vi "Adaptive Filter sim_edit_JMS.vi"() -> ()   [LabVIEW 2013]
uses:
  <vilib>/Utility/file.llb/Read From Spreadsheet File (I64).vi
panel:
  in  "Rescale":bool
  in  "Decimate":bool
  out "Gradients":dbl[][](graph)
  in  "Filter":bool
  in  "Filter Size":i32=100
  out "Weights":dbl[][](graph)
  out "Taps":dbl[][](graph)
  in  "Beta":fxp<+/-,32,-16>=1.000088900582341e-11
  out "ECG Data":dbl[][](graph)
  in  "File Path Control":path=path "C:/Users/pursley/Documents/Projects/NHLBI/Lederman/Testing/2014-03-21/FL1.txt"
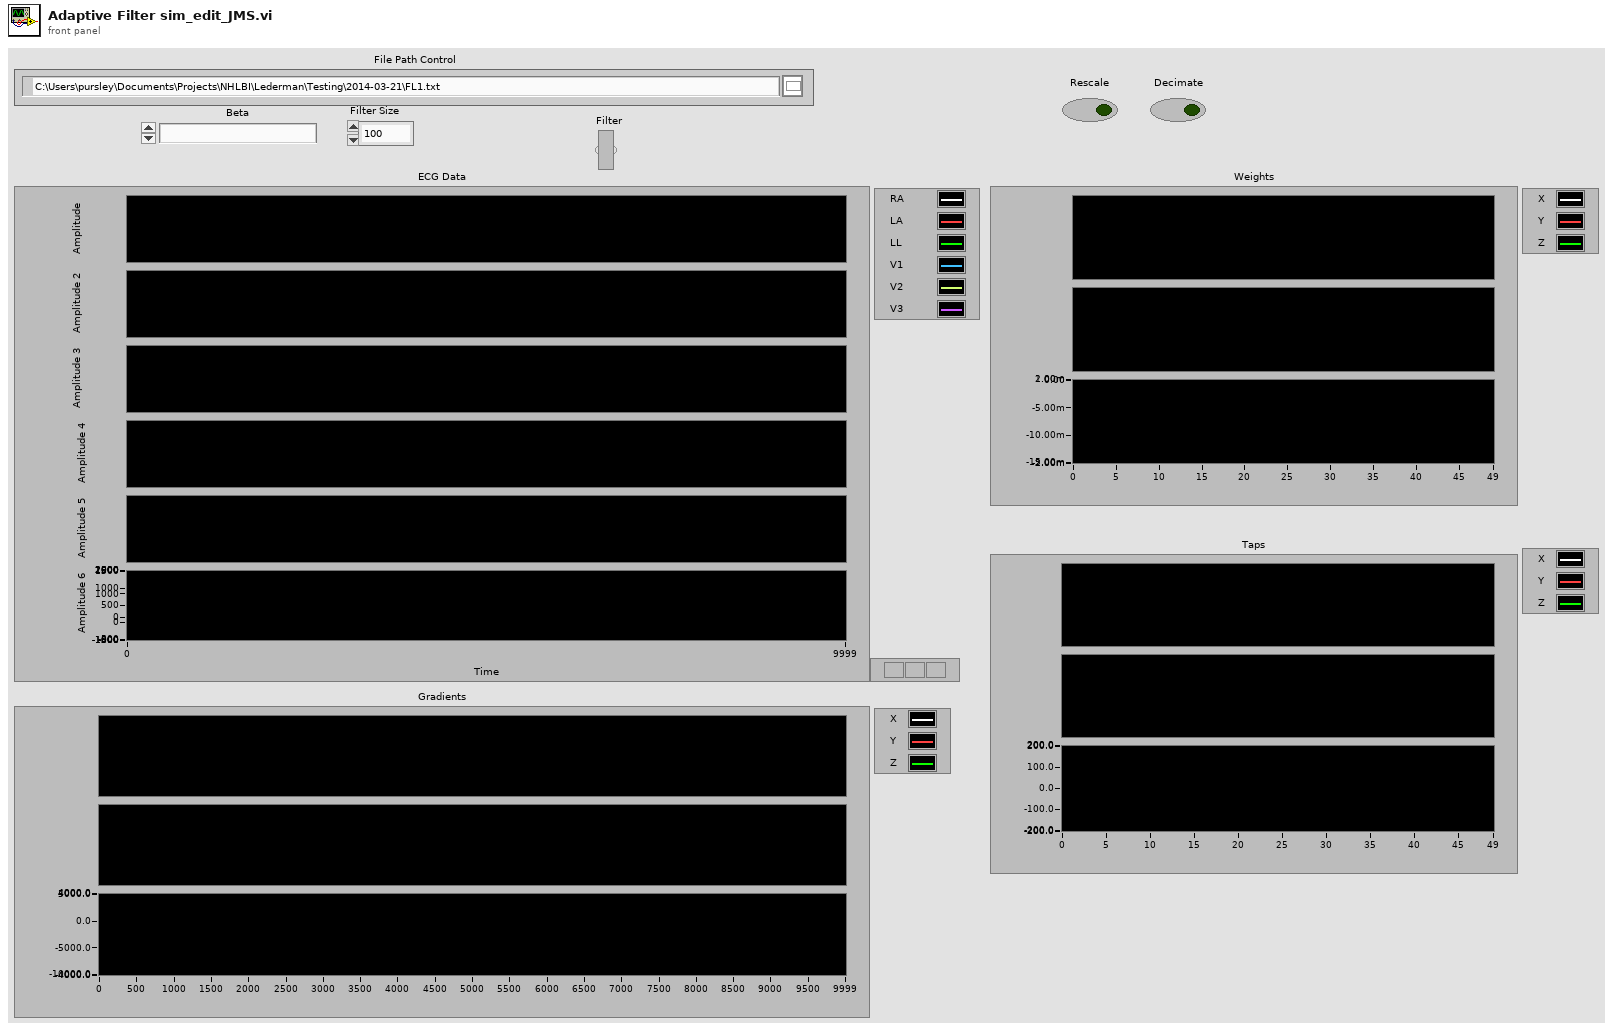
[diagram p1: front panel]
types:
  T1 = cluster{"fixed-point type":fxp<+/-,16,16>, "fixed-point type":fxp<+/-,16,16>, "fixed-point type":fxp<+/-,16,16>}
  T2 = cluster{"fixed-point type":dbl, "fixed-point type":dbl, "fixed-point type":dbl}
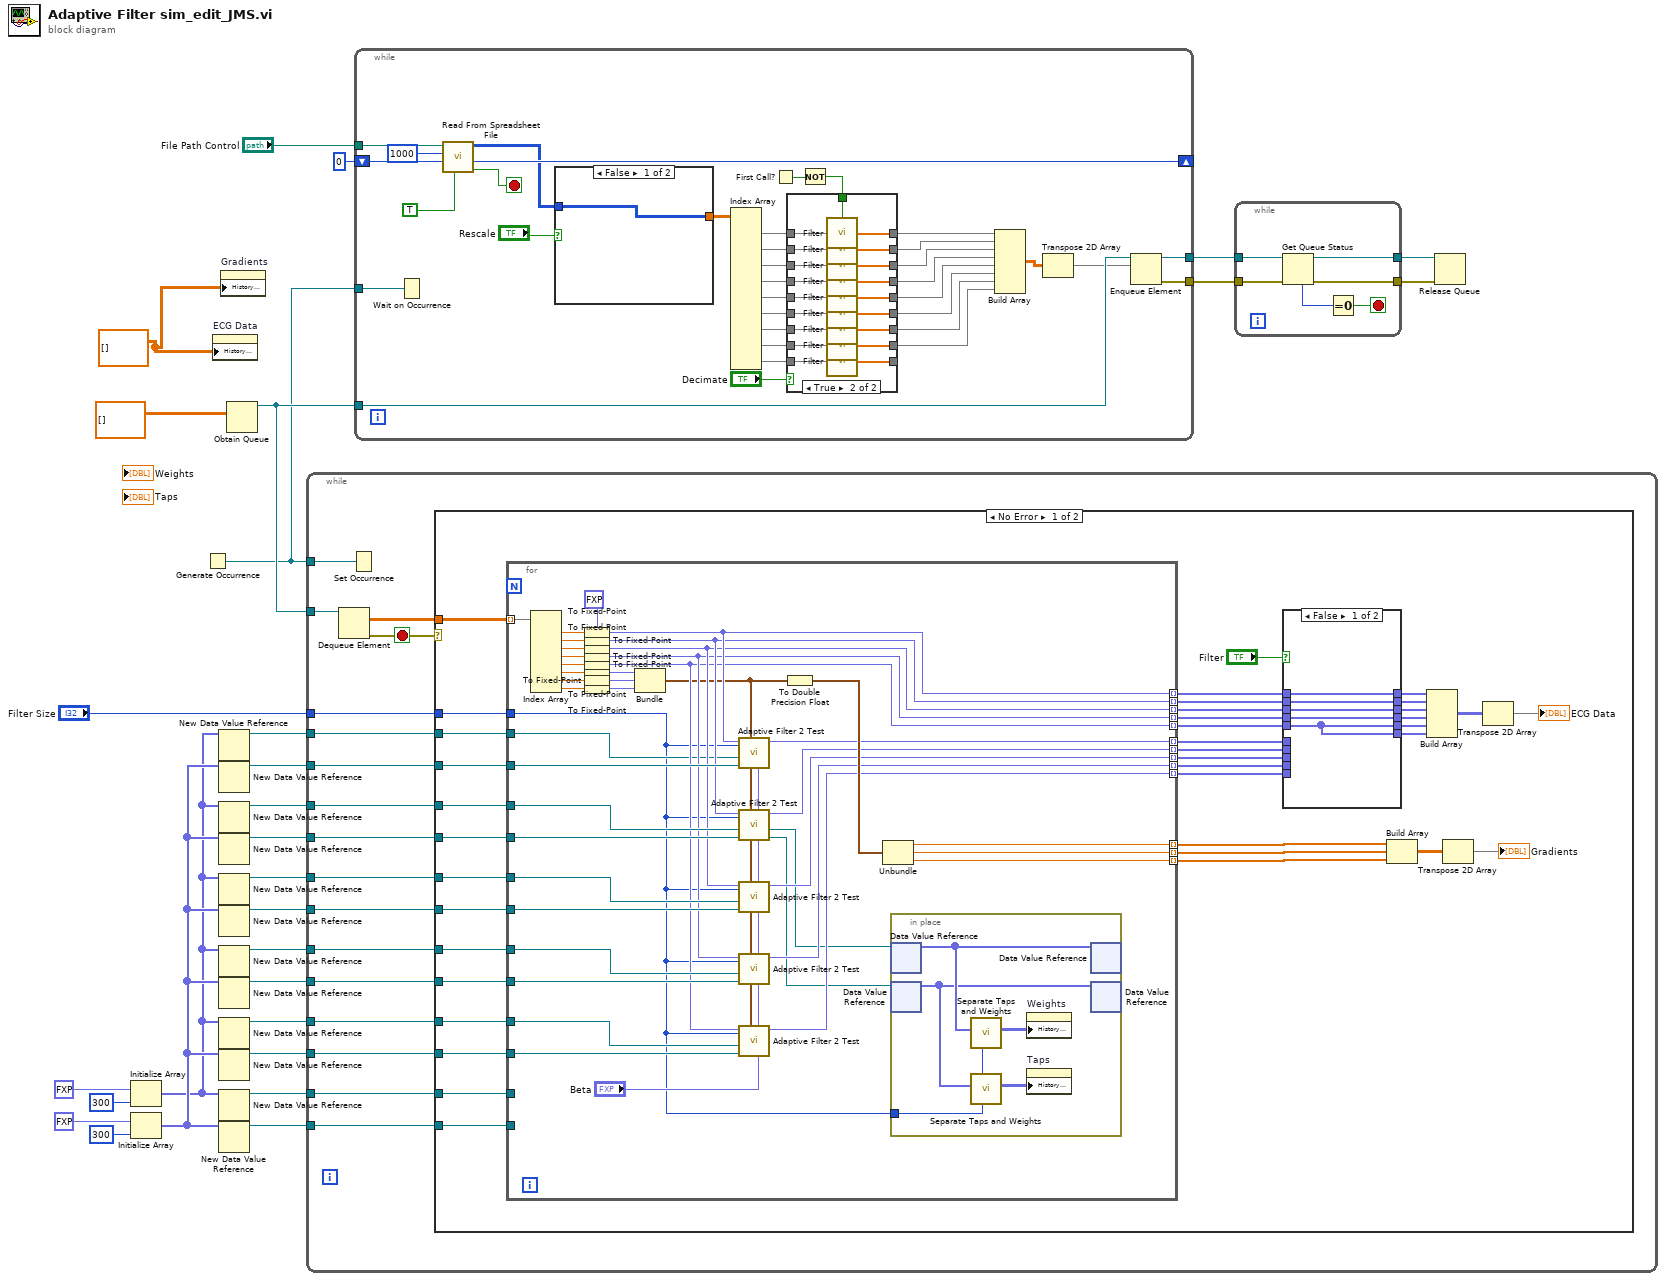
[diagram p0: block diagram]
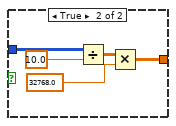
[diagram p4: hidden frame]
diagram:
  w1 = dbl[][] [] ("History Data")
  n1 = Initialize Array(fxp<+/-,24,8> 0.0 ("Z"), 300 ("dimension size")) -> (w8:fxp<+/-,24,8>[])
  n2 = Initialize Array(fxp<+/-,16,16> 0.0 ("Z"), 300 ("dimension size")) -> (w11:fxp<+/-,16,16>[])
  n3 = Generate Occurrence() -> (w2:refnum<k4>)
  n4 = property on="ECG Data" class="WFChart (strict)"("History Data"=w1) -> ()  [unwired: 2 in, 2 out]
  n5 = New Data Value Reference(data value=w8) -> (data value reference=w25:refnum<data-value>)  [unwired: 1 in, 1 out]
  n6 = New Data Value Reference(data value=w11) -> (data value reference=w24:refnum<data-value>)  [unwired: 1 in, 1 out]
  n7 = New Data Value Reference(data value=w8) -> (data value reference=w22:refnum<data-value>)  [unwired: 1 in, 1 out]
  n8 = New Data Value Reference(data value=w11) -> (data value reference=w23:refnum<data-value>)  [unwired: 1 in, 1 out]
  n9 = New Data Value Reference(data value=w8) -> (data value reference=w20:refnum<data-value>)  [unwired: 1 in, 1 out]
  n10 = New Data Value Reference(data value=w11) -> (data value reference=w21:refnum<data-value>)  [unwired: 1 in, 1 out]
  n11 = New Data Value Reference(data value=w8) -> (data value reference=w18:refnum<data-value>)  [unwired: 1 in, 1 out]
  n12 = New Data Value Reference(data value=w11) -> (data value reference=w19:refnum<data-value>)  [unwired: 1 in, 1 out]
  n13 = New Data Value Reference(data value=w8) -> (data value reference=w16:refnum<data-value>)  [unwired: 1 in, 1 out]
  n14 = New Data Value Reference(data value=w11) -> (data value reference=w17:refnum<data-value>)  [unwired: 1 in, 1 out]
  n15 = New Data Value Reference(data value=w8) -> (data value reference=w14:refnum<data-value>)  [unwired: 1 in, 1 out]
  n16 = New Data Value Reference(data value=w11) -> (data value reference=w15:refnum<data-value>)  [unwired: 1 in, 1 out]
  n17 = property on="Gradients" class="WFChart (strict)"("History Data"=w1) -> ()  [unwired: 2 in, 2 out]
  n18 = Obtain Queue(element data type=dbl[][] [] ("History Data")) -> (queue out=w26:refnum<queue>)  [unwired: 4 in, 2 out]
  n19 = while {
    tunnel: w26 -> [w30]
    tunnel: w25 -> [w44]
    tunnel: w24 -> [w43]
    tunnel: w23 -> [w42]
    tunnel: w22 -> [w41]
    tunnel: w21 -> [w40]
    tunnel: w20 -> [w39]
    tunnel: w19 -> [w38]
    tunnel: w18 -> [w37]
    tunnel: w17 -> [w36]
    tunnel: w16 -> [w35]
    tunnel: w15 -> [w34]
    tunnel: w14 -> [w33]
    tunnel: "Filter Size" -> [w32]
    tunnel: w2 -> [w31]
    stop <- w46 stop-if-true
    n20 = Dequeue Element(queue=w30) -> (element=w45:dbl[][], error out=w46:errorcluster)  [unwired: 2 in, 2 out]
    n21 = Set Occurrence(w31) -> ()
    n22 = case shown="No Error" w46 {
      tunnel: w45 -> [w84 _]
      tunnel: w44 -> [w83 _]
      tunnel: w43 -> [w82 _]
      tunnel: w42 -> [w81 _]
      tunnel: w41 -> [w80 _]
      tunnel: w40 -> [w79 _]
      tunnel: w39 -> [w78 _]
      tunnel: w38 -> [w77 _]
      tunnel: w37 -> [w76 _]
      tunnel: w36 -> [w75 _]
      tunnel: w35 -> [w74 _]
      tunnel: w34 -> [w73 _]
      tunnel: w33 -> [w72 _]
      tunnel: w32 -> [w69 _]
      frame No Error {
        n23 = for {
          tunnel: w84 -> [w136] mode=indexing
          tunnel: w83 -> [w102]
          tunnel: w82 -> [w126]
          tunnel: w81 -> [w125]
          tunnel: w80 -> [w124]
          tunnel: w79 -> [w123]
          tunnel: w78 -> [w122]
          tunnel: w77 -> [w121]
          tunnel: w76 -> [w120]
          tunnel: w75 -> [w118]
          tunnel: w74 -> [w117]
          tunnel: w73 -> [_]
          tunnel: w72 -> [_]
          tunnel: [w115] -> w68 mode=indexing
          tunnel: [w114] -> w67 mode=indexing
          tunnel: [w113] -> w66 mode=indexing
          tunnel: [w112] -> w65 mode=indexing
          tunnel: [w111] -> w64 mode=indexing
          tunnel: [w110] -> w63 mode=indexing
          tunnel: [w109] -> w62 mode=indexing
          tunnel: [w108] -> w61 mode=indexing
          tunnel: [w107] -> w60 mode=indexing
          tunnel: [w106] -> w59 mode=indexing
          tunnel: [w105] -> w51 mode=indexing
          tunnel: [w104] -> w50 mode=indexing
          tunnel: [w103] -> w49 mode=indexing
          tunnel: w69 -> [w100]
          w130 = fxp<+/-,16,16> 0.0 ("fixed-point type")
          n24 = Index Array(array=w136) -> (element #1=w135:dbl, element #2=w134:dbl, element #3=w133:dbl, element #4=w132:dbl, element #5=w131:dbl, element #6=w99:dbl, element #7=w98:dbl, element #8=w97:dbl)  [unwired: 8 in]
          n25 = To Fixed-Point(fixed-point type=w130, number=w135) -> (fixed-point=w115:fxp<+/-,16,16>)
          n26 = To Fixed-Point(fixed-point type=w130, number=w134) -> (fixed-point=w114:fxp<+/-,16,16>)
          n27 = To Fixed-Point(fixed-point type=w130, number=w133) -> (fixed-point=w113:fxp<+/-,16,16>)
          n28 = To Fixed-Point(fixed-point type=w130, number=w132) -> (fixed-point=w112:fxp<+/-,16,16>)
          n29 = To Fixed-Point(fixed-point type=w130, number=w131) -> (fixed-point=w111:fxp<+/-,16,16>)
          n30 = To Fixed-Point(fixed-point type=w130, number=w99) -> (fixed-point=w129:fxp<+/-,16,16>)
          n31 = To Fixed-Point(fixed-point type=w130, number=w98) -> (fixed-point=w128:fxp<+/-,16,16>)
          n32 = To Fixed-Point(fixed-point type=w130, number=w97) -> (fixed-point=w127:fxp<+/-,16,16>)
          n33 = Bundle("fixed-point type"=w129, "fixed-point type"=w128, "fixed-point type"=w127) -> (w101:T1)  [unwired: 1 in]
          n34 = call "Adaptive Filter 2 Test.vi"("Beta"="Beta", "Noise"=w101, "Filter Size"=w100, "Taps In"=w126, "Weights In"=w102, "Input"=w115) -> ("Error Out"=w110:fxp<+/-,16,16>)  [unwired: 3 in, 2 out]
          n35 = call "Adaptive Filter 2 Test.vi"("Beta"="Beta", "Noise"=w101, "Filter Size"=w100, "Taps In"=w125, "Weights In"=w124, "Input"=w114) -> ("Taps Out"=w96:refnum<data-value>, "Weights Out"=w95:refnum<data-value>, "Error Out"=w109:fxp<+/-,16,16>)  [unwired: 3 in]
          n36 = call "Adaptive Filter 2 Test.vi"("Beta"="Beta", "Noise"=w101, "Filter Size"=w100, "Taps In"=w123, "Weights In"=w122, "Input"=w113) -> ("Error Out"=w108:fxp<+/-,16,16>)  [unwired: 3 in, 2 out]
          n37 = call "Adaptive Filter 2 Test.vi"("Beta"="Beta", "Noise"=w101, "Filter Size"=w100, "Taps In"=w121, "Weights In"=w120, "Input"=w112) -> ("Error Out"=w107:fxp<+/-,16,16>)  [unwired: 3 in, 2 out]
          n38 = call "Adaptive Filter 2 Test.vi"("Beta"="Beta", "Noise"=w101, "Filter Size"=w100, "Taps In"=w118, "Weights In"=w117, "Input"=w111) -> ("Error Out"=w106:fxp<+/-,16,16>)  [unwired: 3 in, 2 out]
          n39 = To Double Precision Float(number=w101) -> (double precision float=w116:T2)
          n40 = Unbundle(w116) -> ("fixed-point type"=w105:dbl, "fixed-point type"=w104:dbl, "fixed-point type"=w103:dbl)
          n41 = in-place {
            in-place-border: w100 -> [w139]
            n42 = in-place-dvr #1(w95) -> (w141:fxp<+/-,24,8>[])  [unwired: 1 out]
            n43 = in-place-dvr #2(w96) -> (w140:fxp<+/-,16,16>[])  [unwired: 1 out]
            n44 = call "Separate Taps and Weights.vi"("Filter Size"=w139, "Array in"=w141) -> ("Array out"=w138:fxp<+/-,24,8>[][])  [unwired: 9 in]
            n45 = call "Separate Taps and Weights.vi"("Filter Size"=w139, "Array in"=w140) -> ("Array out"=w137:fxp<+/-,24,8>[][])  [unwired: 9 in]
            n46 = property on="Weights" class="WFChart (strict)"("History Data"=w138) -> ()  [unwired: 2 in, 2 out]
            n47 = property on="Taps" class="WFChart (strict)"("History Data"=w137) -> ()  [unwired: 2 in, 2 out]
            n48 = in-place-dvr #1(w141) -> ()  [unwired: 2 out]
            n49 = in-place-dvr #2(w140) -> ()  [unwired: 2 out]
          }
        }
        n50 = case shown="False" "Filter" {
          tunnel: w68 -> [w89 _]
          tunnel: w67 -> [w88 _]
          tunnel: w66 -> [w87 _]
          tunnel: w65 -> [w86 _]
          tunnel: w64 -> [w85 _]
          tunnel: w63 -> [_ w94]
          tunnel: w62 -> [_ w93]
          tunnel: w61 -> [_ w92]
          tunnel: w60 -> [_ w91]
          tunnel: w59 -> [_ w90]
          tunnel: [w89 w94] -> w58
          tunnel: [w88 w93] -> w57
          tunnel: [w87 w92] -> w56
          tunnel: [w86 w91] -> w55
          tunnel: [w85 w90] -> w54
          tunnel: [w85 w90] -> w47
          frame False {
          }
          frame True {
          }
        }
        n51 = Build Array(w51, w50, w49) -> (w52:dbl[][])
        n52 = Build Array(w58, w57, w56, w55, w54, w47) -> (w71:fxp<+/-,16,16>[][])
        n53 = Transpose 2D Array(2D array=w52) -> (transposed array=→"Gradients":dbl[][])
        n54 = Transpose 2D Array(2D array=w71) -> (transposed array=→"ECG Data":fxp<+/-,16,16>[][])
      }
      frame Error {
      }
    }
  }
  n55 = while {
    tunnel: "File Path Control" -> [w176]
    shift-right: [w174] -> _
    shift-left: 0 ("mark after read (chars.)") -> [w173]
    tunnel: w26 -> [w150]
    tunnel: [w149] -> w7
    tunnel: [w146] -> w5
    tunnel: w2 -> [w145]
    stop <- w171 stop-if-true
    n56 = Wait on Occurrence(2:w145) -> ()  [unwired: 2 in, 1 out]
    n57 = call-poly <vilib>:"Read From Spreadsheet File.vi"("transpose (no:F)"=TRUE, "start of read offset (chars.:0)"=w173, "number of rows (all:-1)"=1000, "file path (dialog if empty)"=w176) -> ("EOF?"=w171:bool, "mark after read (chars.)"=w174:i32, "all rows"=w170:i64[][])  [unwired: 3 in, 2 out]
    n58 = case shown="False" "Rescale" {
      tunnel: w170 -> [w177 w182]
      tunnel: [w177 w178] -> w169
      frame False {
      }
      frame True {
        n59 = Divide(x=w182, y=10.0) -> (x/y=w180:dbl[][])
        n60 = Multiply(x=w180, y=32768.0) -> (x*y=w178:dbl[][])
      }
    }
    n61 = Index Array(array=w169) -> (element #1=w168:dbl[], element #2=w166:dbl[], element #3=w165:dbl[], element #4=w164:dbl[], element #5=w163:dbl[], element #6=w162:dbl[], element #7=w161:dbl[], element #8=w160:dbl[], element #9=w159:dbl[])  [unwired: 18 in]
    n62 = First Call?() -> (First Call?: T/F=w167:bool)
    n63 = Not(x=w167) -> (.not. x?=w158:bool)
    n64 = case shown="True" "Decimate" {
      tunnel: w168 -> [w191 w210]
      tunnel: w166 -> [w190 w209]
      tunnel: w165 -> [w189 w208]
      tunnel: w164 -> [w188 w207]
      tunnel: w163 -> [w187 w206]
      tunnel: w162 -> [w186 w205]
      tunnel: w161 -> [w185 w204]
      tunnel: w160 -> [w184 w203]
      tunnel: w159 -> [w183 w202]
      tunnel: w158 -> [_ w201]
      tunnel: [w191 w200] -> w157
      tunnel: [w190 w199] -> w142
      tunnel: [w189 w198] -> w156
      tunnel: [w188 w197] -> w155
      tunnel: [w187 w196] -> w154
      tunnel: [w186 w195] -> w153
      tunnel: [w185 w194] -> w152
      tunnel: [w184 w193] -> w151
      tunnel: [w183 w192] -> _
      frame False {
      }
      frame True {
        n65 = call "Filter.vi"("Array"=w210, "init/cont (init:F)"=w201) -> ("Decimated Array"=w200:dbl[])
        n66 = call "Filter.vi"("Array"=w209, "init/cont (init:F)"=w201) -> ("Decimated Array"=w199:dbl[])
        n67 = call "Filter.vi"("Array"=w208, "init/cont (init:F)"=w201) -> ("Decimated Array"=w198:dbl[])
        n68 = call "Filter.vi"("Array"=w207, "init/cont (init:F)"=w201) -> ("Decimated Array"=w197:dbl[])
        n69 = call "Filter.vi"("Array"=w206, "init/cont (init:F)"=w201) -> ("Decimated Array"=w196:dbl[])
        n70 = call "Filter.vi"("Array"=w205, "init/cont (init:F)"=w201) -> ("Decimated Array"=w195:dbl[])
        n71 = call "Filter.vi"("Array"=w204, "init/cont (init:F)"=w201) -> ("Decimated Array"=w194:dbl[])
        n72 = call "Filter.vi"("Array"=w203, "init/cont (init:F)"=w201) -> ("Decimated Array"=w193:dbl[])
        n73 = call "Filter.vi"("Array"=w202, "init/cont (init:F)"=w201) -> ("Decimated Array"=w192:dbl[])
      }
    }
    n74 = Build Array(w157, w142, w156, w155, w154, w153, w152, w151) -> (w148:dbl[][])
    n75 = Transpose 2D Array(2D array=w148) -> (transposed array=w147:dbl[][])
    n76 = Enqueue Element(queue=w150, element=w147) -> (queue out=w149:refnum<queue>, error out=w146:errorcluster)  [unwired: 2 in, 1 out]
  }
  n77 = while {
    tunnel: w7 -> [w216]
    tunnel: [w215] -> w6
    tunnel: w5 -> [w214]
    tunnel: [w213] -> w4
    stop <- w211 stop-if-true
    n78 = Get Queue Status(queue=w216, error in (no error)=w214) -> (queue out=w215:refnum<queue>, error out=w213:errorcluster, # elements in queue=w212:i32)  [unwired: 1 in, 5 out]
    n79 = Equal To 0?(x=w212) -> (x = 0?=w211:bool)
  }
  n80 = Release Queue(queue=w6, error in (no error)=w4) -> ()  [unwired: 1 in, 3 out]
